vi "Untitled 20 (SubVI).vi"(6 "pulse shaping filter (none)":T1(ring), 7 "carrier frequency (Hz)":dbl min=-0.5 max=0.5 format="%.2f", 9 "Ts":dbl, 10 "Fs":dbl, 11 "см. 1.5 in":dbl[](array[numeric])) -> (1 "Numeric":i32, 2 "passband waveform":waveform(dbl), 3 "Array":waveform(dbl)[](array[waveform]), 4 "Rs":dbl)   [LabVIEW 2017]
uses:
  <vilib>/addons/Modulation/Analog/support/mod_Set Error Source.vi
  <vilib>/addons/Modulation/Digital/Support/Common/Validators/mod_Generate Filter Coefficients Validate.vi
  <vilib>/addons/Modulation/Digital/General/subVIs/mod_Generate Filter Coefficients.vi
  <vilib>/addons/Modulation/Digital/General/MT Generate ASK system parameters (M).vi
  <vilib>/addons/Modulation/Analog/MT Upconvert Baseband (Real).vi
  <vilib>/addons/Modulation/niDMT.lvlib
  <vilib>/addons/Modulation/niAMT.lvlib
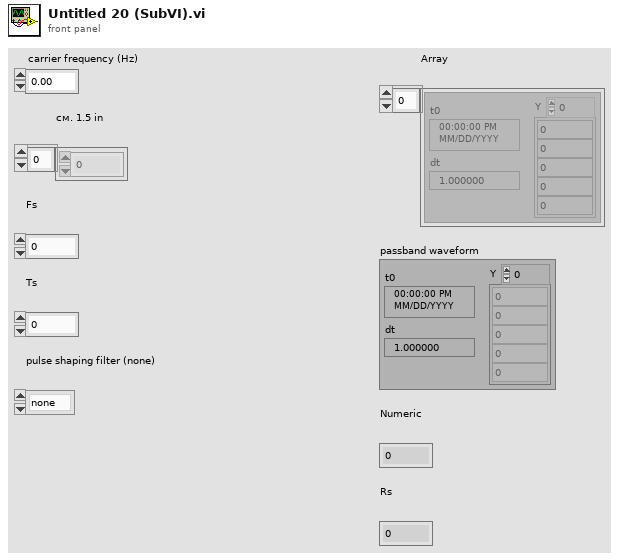
[diagram p1: front panel]
types:
  T1 = enum16{"none", "Raised Cosine", "Root Raised Cos", "Gaussian"}
  T2 = enum16{"FSK", "PSK", "QAM", "MSK", "PAM", "ASK", "CPM"}
  T3 = cluster{"samples per symbol (16)":i32, "symbol map":cdb[]}
  T4 = typedef "niAMT.lvlib/Complex Data Waveform.ctl" = cluster{"t0":dbl, "dt":dbl, "Y":cdb[]}
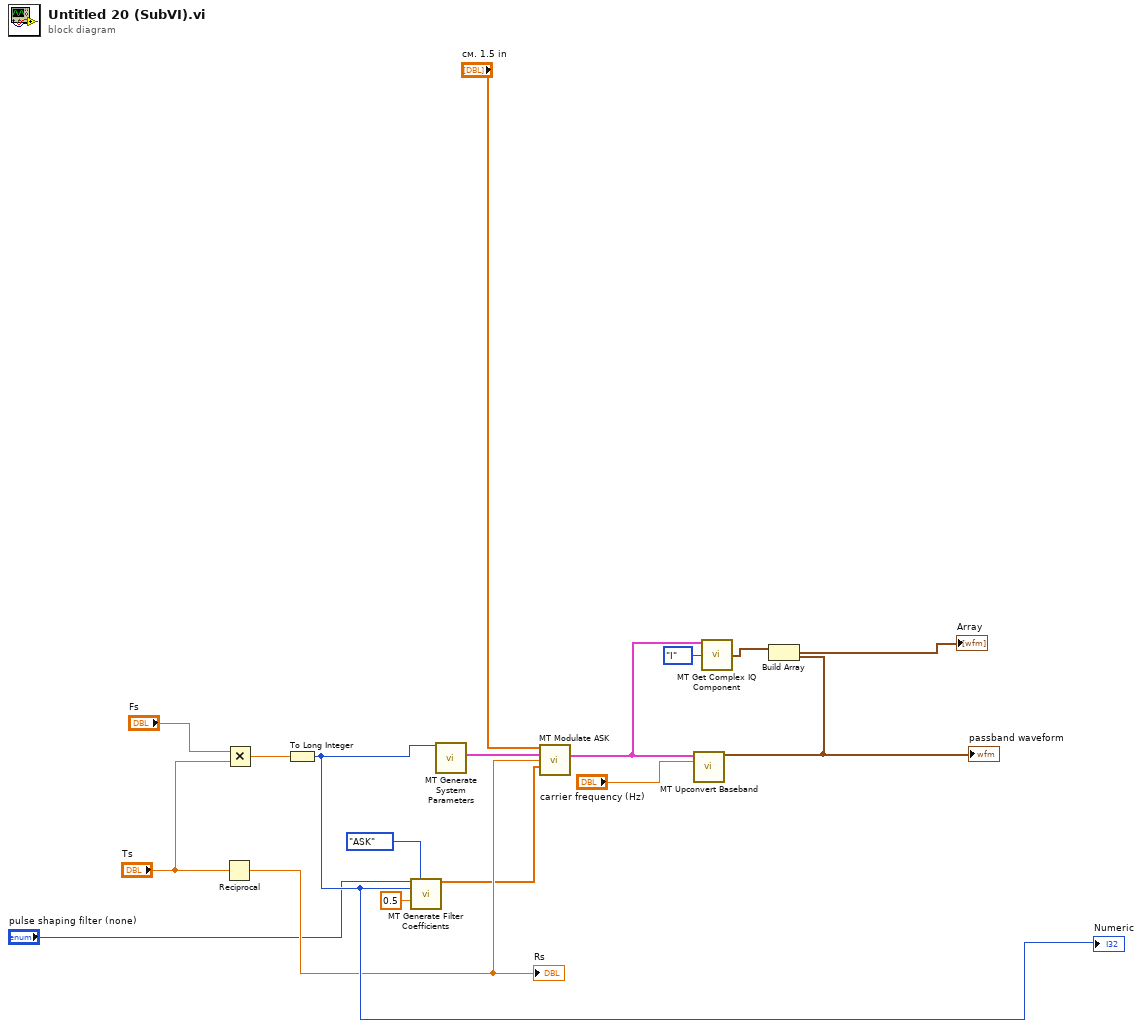
[diagram p0: block diagram]
diagram:
  n1 = Reciprocal(x="Ts") -> (1/x=w11:dbl)
  "Rs" <- w11
  n2 = Multiply(x="Fs", y="Ts") -> (x*y=w3:dbl)
  n3 = To Long Integer(number=w3) -> (32bit integer=w15:i32)
  "Numeric" <- w15
  n4 = call <vilib>:"MT Generate Filter Coefficients.vi"("pulse shaping filter (none)"="pulse shaping filter (none)", "modulation type"=T2."ASK", "pulse shaping samples per symbol (16)"=w15, "filter parameter"=0.5) -> ("pulse shaping filter coefficients"=w6:dbl[])  [unwired: 9 in, 2 out]
  n5 = call-poly <vilib>:"MT Generate System Parameters.vi"("samples per symbol (16)"=w15) -> ("ASK system parameters"=w7:T3)  [unwired: 12 in, 2 out]
  n6 = call <vilib>:"MT Modulate ASK.vi"("input bit stream"="см. 1.5 in", "ASK system parameters"=w7, "symbol rate (Hz)"=w11, "pulse shaping filter coefficients"=w6) -> ("output complex waveform"=w17:T4)  [unwired: 9 in, 2 out]
  n7 = call-poly <vilib>:"MT Upconvert Baseband.vi"("baseband waveform (complex)"=w17, "carrier frequency (Hz)"="carrier frequency (Hz)") -> ("passband waveform"=w14:waveform(dbl))  [unwired: 12 in, 1 out]
  "passband waveform" <- w14
  n8 = call <vilib>:"MT Get Complex IQ Component.vi"("IQ data (complex) in"=w17, "component choice"=enum16{"I", "Q", "Magnitude", "Phase"}."I") -> ("CE component"=w12:waveform(dbl))  [unwired: 11 in, 2 out]
  n9 = Build Array(w12, w14) -> (→"Array":waveform(dbl)[])
